vi "UHR-Fleezers Control (host) - Lorentz v3.vi"() -> ()   [LabVIEW 2014] (continued)
      n899 = xnode "Read/Write Control"("FPGA VI Reference In"=w1386, "error in"=w1384, "Invert GI"=w1380, "Invert GI 2"=w1380, "Invert RI"=w1380, "Invert RI 2"=w1380, "Operating Mode"=w1378, "Operating Mode 2"=w1378, "Red Laser Operating Mode"=w1378, "RI Operating Mode 2"=w1378, "P3"=w1410, "I3"=w1411, "D3"=w1412, "Green FB Setpoint"=w1396, "Green FB On/Off"="Green FB On/Off", "Current Out"=w1393, "Green int current ON count adj"="Green int current ON count adj", "Trap Pos FB Monitor T1 or T2"=w1397, "Trap Pos FB Negate Action"=w1398, "Trap Pos. FB Offset Factor"=w1399, "Trap Pos. FB Mult Factor"=w1400, "Force feedback"=FALSE, "AI1 X Scale"=w1402, "Trap Pos to FIFO"=TRUE, "Trap Pos FB Int Count"=w1404, "TTrig Negate Pos"=w1405, "FB Trig Integrate"="FB Trig Integrate", "Diff FB Measurement?"=w1407, "Negate Diff?"="Negate Diff?", "Trap pos. FB Range"=w1381, "Trap Pos. FB Gains"=w1382, "Red FB Setpoint"=w1416, "RI Current Out"=w1420, "P4"=w1422, "I4"=w1423, "D4"=w1424, "Red FB On/Off"="Red FB On/Off", "Dynamic Force FB (Ronen)"=w1383) -> ("error out"=w1385:errorcluster)  [unwired: 1 out]
      n900 = local write "FPGA error out"(w1385) -> ()
    }
    frame #3 {
      # "Initialize more settings. Should stop using event loops to initialize."
      # "What are these?"
      n901 = local write "Offset (nm)"(0.0 ("Offset (nm)")) -> ()
      n902 = local write "Bead Mean (nm)"(0.0 ("Bead Mean (nm)")) -> ()
      n903 = stacked-sequence {
        frame #0 {
          w1428 = T43."empty" ("mode")
          # "Clear external fluorescence triggering FIFO"
          # "APD loop counts"
          # "Fluorescence loop counts (rates)"
          n904 = local read "APD Integration Time (s)"() -> (w1430:dbl)
          n905 = local read "Interlace ON count"() -> (w1431:u16)
          n906 = call "Smart Buffer (DBL) 1.vi"("mode"=w1428) -> ()  [unwired: 5 in, 6 out]
          n907 = call "Smart Buffer (DBL) 2.vi"("mode"=w1428) -> ()  [unwired: 5 in, 6 out]
          n908 = property on="APD Integration Time (s)" class="DigNum (strict)"("Val(Sgnl)"=w1430) -> ()  [unwired: 2 in, 2 out]
          n909 = property on="Interlace ON count" class="DigNum (strict)"("Val(Sgnl)"=w1431) -> ()  [unwired: 2 in, 2 out]
          "Number of APDs" <- 3.0 ("Number of APDs")
        }
        frame #1 {
          # "Number of APDs affects\nAPD DMA transfer"
          # "General settings for all lasers:"
          # "And includes all laser\nON/OFF settings"
          # "Fluorescent lasers settings:"
          # "Blue laser settings:"
          n910 = local read "Laser interlacing mode"() -> (w1433:enum32{"Laser ON", "Laser OFF", "Interlace"})
          n911 = local read "Invert laser interlacing"() -> (w1432:bool)
          n912 = local read "Blue FB On/Off"() -> (w1434:bool)
          n913 = property on="Blue FB On/Off" class="Bool (strict)"("Val(Sgnl)"=w1434) -> ()  [unwired: 2 in, 2 out]
          n914 = property on="Invert laser interlacing" class="Bool (strict)"("Val(Sgnl)"=w1432) -> ()  [unwired: 2 in, 2 out]
          n915 = property on="Laser interlacing mode" class="RadioBtnsControl (strict)"("Val(Sgnl)"=w1433) -> ()  [unwired: 2 in, 2 out]
        }
        frame #2 {
          w1435 = path "C:/Home/Bustamante Lab/Comstock-LabView-Link.udl" ("connection information")
          # "Database link changed by Ronen - not clear if it matter for the program."
          # "Initialize the database connection"
          n916 = disable-structure shown="Disabled" {
            disable-tunnel: [w1438 _] -> w1436
            disable-tunnel: w1435 -> [w1437 _]
            frame Disabled {
              n917 = call-poly <vilib>:"DB Tools Open Connection.vi"("connection information"=w1437) -> ("connection reference"=w1438:T25)  [unwired: 7 in, 1 out]
            }
            frame Enabled {
            }
          }
          "connection reference" <- w1436
          n918 = local write "connection reference"(w1436) -> ()
          n919 = local write "Database link"(w1435) -> ()
        }
        frame #3 {
          # "Load active calibration to fpga"
          n920 = local read "Base N trap periods"() -> (w1440:u32)
          n921 = local read "T1 Osc Enable"() -> (w1439:bool)
          n922 = property on="T1 Osc Enable" class="Bool (strict)"("Val(Sgnl)"=w1439) -> ()  [unwired: 2 in, 2 out]
          n923 = property on="Base N trap periods" class="DigNum (strict)"("Val(Sgnl)"=w1440) -> ()  [unwired: 2 in, 2 out]
        }
      }
    }
    frame #4 {
      # "Set FIFO size and run FPGA"
      n924 = local read "FPGA error out"() -> (w1442:errorcluster)
      n925 = xnode "Invoke Method"("FPGA VI Reference In"=w1443, "error in"=w1442, "Requested Depth"="Trap AI FIFO Depth") -> ("FPGA VI Reference Out"=w1447:T36, "error out"=w1448:errorcluster)  [unwired: 1 out]
      n926 = xnode "Invoke Method"("FPGA VI Reference In"=w1447, "error in"=w1448, "Requested Depth"="Trap Position FIFO Depth") -> ("FPGA VI Reference Out"=w1445:T36, "error out"=w1444:errorcluster)  [unwired: 1 out]
      n927 = xnode "Invoke Method"("FPGA VI Reference In"=w1445, "error in"=w1444) -> ("error out"=w1441:errorcluster)  [unwired: 1 in, 1 out]
      n928 = local write "FPGA error out"(w1441) -> ()
    }
    frame #5 {
      # "Adjust FPGA timing loop phases"
      n929 = flat-sequence "Initial FPGA Loop Relative Phase Adjustment" {
        tunnel: "Initial Phase Adjustment (AI1)" -> [w1482]
        tunnel: "Initial Phase Adjustment (GI)" -> [w1481]
        tunnel: "Initial Phase Adj. (MCL)" -> [w1480]
        tunnel: [w1483] -> w1467
        tunnel: [w1479] -> w1466
        tunnel: "Initial Phase Adjustment (APD Acq)" -> [w1478]
        tunnel: "Initial Phase Adjustment (APD 1 Gate)" -> [w1477]
        tunnel: "Initial Phase Adjustment (Green FB)" -> [w1476]
        tunnel: "Initial Phase Adjustment (GI) 2" -> [w1475]
        tunnel: "Initial Phase Adjustment (APD 2 Gate)" -> [w1474]
        tunnel: "Initial Phase Adjustment (RI)" -> [w1473]
        tunnel: "Initial Phase Adjustment (BI DO)" -> [w1472]
        tunnel: "Initial Phase Adjustment (BI AO)" -> [w1471]
        tunnel: "Initial Phase Adjustment (APD 3 Gate)" -> [w1470]
        tunnel: w1452 -> [w1469]
        tunnel: w1467 -> [w1485]
        tunnel: [w1486] -> w1465
        tunnel: w1466 -> [w1486]
        tunnel: [w1485] -> w1464
        tunnel: w1465 -> [w1490]
        tunnel: w1464 -> [w1489]
        tunnel: [w1487] -> w1451
        frame #0 {
          n930 = local read "FPGA error out"() -> (w1468:errorcluster)
          n931 = xnode "Read/Write Control"("FPGA VI Reference In"=w1469, "error in"=w1468, "Phase count adjustment"=w1482, "Phase count adjustment (GI)"=w1481, "Phase count adjustment (MCL)"=w1480, "Phase Count Adjustment (APD Acq)"=w1478, "Phase count adjustment (APD 1 Gate)"=w1477, "Phase count adjustment (APD 2 Gate)"=w1474, "Phase count adjustment (Green FB)"=w1476, "Phase count adjustment (GI) 2"=w1475, "Phase count adjustment (RI)"=w1473, "Phase count adjustment (BI AO)"=w1471, "Phase count adjustment (BI D)"=w1472, "Phase count adjustment (APD 3 Gate)"=w1470) -> ("FPGA VI Reference Out"=w1479:T36, "error out"=w1483:errorcluster)
        }
        frame #1 {
          n932 = Wait (ms)(milliseconds to wait=u32 100) -> ()  [unwired: 1 out]
        }
        frame #2 {
          w1488 = TRUE
          n933 = xnode "Read/Write Control"("FPGA VI Reference In"=w1490, "error in"=w1489, "+ phase"=w1488, "+ phase (GI)"=w1488, "+ phase (MCL)"=w1488, "+ phase (APD Acq)"=w1488, "+ phase (APD 1 Gate)"=w1488, "+ phase (APD 2 Gate)"=w1488, "+ phase (Green FB)"=w1488, "+ phase (GI) 2"=w1488, "+ phase (RI)"=w1488, "+ phase (BI AO)"=w1488, "+ phase (BI D)"=w1488, "+ phase (APD 3 Gate)"=w1488) -> ("error out"=w1487:errorcluster)  [unwired: 1 out]
        }
      }
      n934 = local write "FPGA error out"(w1451) -> ()
    }
    frame #6 {
      w1504 = 6.0  # clock mult.
      w1503 = 49152000.0  # TCXO frequ.
      w1508 = 6.0  # clock mult.
      w1509 = 49152000.0  # TCXO frequ.
      # "Added by ronen - definition of \nlimit frequencies when using dynamic feedback"
      # "Initialize trap RF synth board and set initial frequencies and amplitudes"
      n935 = local read "FPGA error out"() -> (w1518:errorcluster)
      n936 = call "Initialize RF boards - interlace 3.vi"("error in"=w1518, "FPGA VI Reference In"=w1519) -> ("error out"=w1520:errorcluster, "FPGA VI Reference Out"=w1540:T36)
      n937 = call "set RF board frequency - interlace.vi"("Board 2 Frequency Limits"=w1515, "Board 1 Frequency Limits"=w1496, "error in"=w1520, "FPGA VI Reference In"=w1540, "Board 2 Frequency 3 (MHz)"="BD 2 Frequency 3 (MHz)", "Board 1 Frequency 3 (MHz)"="BD 1 Frequency 3 (MHz)", "Board 2 Frequency 2 (MHz)"="BD 2 Frequency 2 (MHz)", "Board 2 Frequency 1 (MHz)"="BD 2 Frequency 1 (MHz)", "Board 1 Frequency 2 (MHz)"="BD 1 Frequency 2 (MHz)", "Board 1 Frequency 1  (MHz)"="BD 1 Frequency 1 (MHz)") -> ("error out"=w1523:errorcluster, "FPGA VI Reference Out"=w1495:T36)
      n938 = Unbundle By Name(w1496) -> ("Maximum"=w1506:dbl, "Minimum"=w1497:dbl)
      n939 = call "set RF board amplitude - interlace.vi"("Board 2 Amplitude Limits"=w1517, "Board 1 Amplitude Limits"=w1516, "error in"=w1523, "FPGA VI Reference In"=w1495, "Board 2 Amplitude 3 (%)"="BD 2 Amplitude 3 (%)", "Board 1 Amplitude 3 (%)"="BD 1 Amplitude 3 (%)", "Board 2 Amplitude 2 (%)"="BD 2 Amplitude 2 (%)", "Board 2 Amplitude 1 (%)"="BD 2 Amplitude 1 (%)", "Board 1 Amplitude 2 (%)"="BD 1 Amplitude 2 (%)", "Board 1 Amplitude 1 (%)"="BD 1 Amplitude 1 (%)") -> ("error out"=w1492:errorcluster)  [unwired: 1 out]
      n940 = Multiply(x=w1497, y=1000000.0) -> (x*y=w1501:dbl)
      n941 = Multiply(x=w1506, y=1000000.0) -> (x*y=w1511:dbl)
      n942 = Scale By Power Of 2(n=48, x=w1501) -> (x*2^n=w1499:dbl)
      n943 = Subtract(x="BD 1 Frequency 1 (MHz)", y="BD 1 Frequency 2 (MHz)") -> (x-y=w1530:dbl)
      n944 = Subtract(x="BD 2 Frequency 1 (MHz)", y="BD 2 Frequency 2 (MHz)") -> (x-y=w1531:dbl)
      n945 = Scale By Power Of 2(n=48, x=w1511) -> (x*2^n=w1513:dbl)
      n946 = Multiply(x=w1503, y=w1504) -> (x*y=w1505:dbl)
      n947 = Multiply(x=w1509, y=w1508) -> (x*y=w1507:dbl)
      n948 = Square(x=w1531) -> (x^2=w1533:dbl)
      n949 = Square(x=w1530) -> (x^2=w1532:dbl)
      n950 = Divide(x=w1499, y=w1505) -> (x/y=w1500:dbl)
      n951 = Divide(x=w1513, y=w1507) -> (x/y=w1512:dbl)
      n952 = Add(x=w1532, y=w1533) -> (x+y=w1534:dbl)
      n953 = To Unsigned Quad Integer(1:w1500) -> (0:w1493:u64)
      n954 = To Unsigned Quad Integer(1:w1512) -> (0:w1494:u64)
      n955 = Square Root(x=w1534) -> (sqrt(x)=w1535:dbl)
      n956 = local write "Trap Delta (MHz)"(w1535) -> ()
      n957 = xnode "Read/Write Control"("FPGA VI Reference In"=w1495, "error in"=w1492, "FB Max Frequency"=w1494, "FB Min frequency"=w1493) -> ("error out"=w1491:errorcluster)  [unwired: 1 out]
      n958 = local write "FPGA error out"(w1491) -> ()
    }
    frame #7 {
      n959 = local read "FPGA error out"() -> (w1542:errorcluster)
      n960 = flat-sequence {
        tunnel: [w1556] -> w1547
        tunnel: [w1555] -> w1546
        tunnel: w1543 -> [w1549]
        tunnel: w1542 -> [w1548]
        tunnel: [w1560] -> w1545
        tunnel: w1547 -> [w1560]
        tunnel: [w1559] -> w1544
        tunnel: w1546 -> [w1559]
        tunnel: w1545 -> [w1568]
        tunnel: w1544 -> [w1567]
        tunnel: [w1562] -> w1541
        frame #0 {
          n961 = xnode "Read/Write Control"("FPGA VI Reference In"=w1549, "error in"=w1548, "Direct RF Box  Communication"=FALSE) -> ("FPGA VI Reference Out"=w1556:T36, "error out"=w1555:errorcluster)
          n962 = local read "Trap 1 (ON/OFF)"() -> (w1550:bool)
          n963 = local write "Saving..."(FALSE ("Saving Data")) -> ()
          n964 = local write "Stop All"(FALSE ("Stop All")) -> ()
          n965 = local write "Index"(1.0 ("Index")) -> ()
          n966 = property on="Trap 1 ON" class="Bool (strict)"("Value"=w1550) -> ()  [unwired: 2 in, 2 out]
          "Manipulating Trap" <- FALSE ("Manipulating Trap")
        }
        frame #1 {
          n967 = local read "Trap 2 (ON/OFF)"() -> (w1558:bool)
          n968 = Wait (ms)(milliseconds to wait=u32 10) -> ()  [unwired: 1 out]
          n969 = property on="Trap 2 ON" class="Bool (strict)"("Val(Sgnl)"=w1558) -> ()  [unwired: 2 in, 2 out]
        }
        frame #2 {
          n970 = local read "Scan Range (nm)"() -> (w1563:dbl)
          n971 = xnode "Read/Write Control"("FPGA VI Reference In"=w1568, "error in"=w1567, "FPGA Controls  RF Box"=TRUE ("Direct RF Box  Communication")) -> ("error out"=w1562:errorcluster)  [unwired: 1 out]
          n972 = call "Update messages.vi"("Message to add"="UHR-Fleezers ready.", "Old message string"="") -> ("New message string"=w1566:string)
          n973 = local write "Messages"(w1566) -> ()
          n974 = property on="Scan Range (nm)" class="DigNum (strict)"("Val(Sgnl)"=w1563) -> ()  [unwired: 2 in, 2 out]
        }
      }
      n975 = local write "FPGA error out"(w1541) -> ()
    }
    frame #8 {
      w1570 = u32 0
      w1576 = cluster{u32, u32} {16777238, 16777238}
      w1571 = 0.0
      n976 = control-ref of="Piezo trap cursor control"() -> (w1572:refnum<vi>)
      n977 = disable-structure shown="Disabled" {
        disable-tunnel: [w1579 _] -> w1578
        frame Disabled {
          n978 = call "hamilton_controller.vi"("action"=T42."CONNECT") -> ("error out"=w1582:errorcluster)  [unwired: 9 in, 1 out]
          n979 = call "hamilton_controller.vi"("error in"=w1582, "action"=T42."INITIALIZE VALVES") -> ("error out"=w1579:errorcluster)  [unwired: 8 in, 1 out]
        }
        frame Enabled {
        }
      }
      n980 = property class="XYGraph (strict)"(reference=w1572, "XScale.Maximum"=10.0, "XScale.Minimum"=w1571, "YScale.Maximum"=w1571, "YScale.Minimum"=-10.0, "Plot Area Colors"=w1576, "Frame Color"=u32 9868950, "XScale.GridColors"=w1576, "YScale.GridColors"=w1576, "Cursor.Cursor Color"=u32 16711680, "Active Cursor"=w1570, "Cursor.CursorMode"=w1570) -> ()  [unwired: 1 in, 2 out]
    }
    frame #9 {
      # "Wait 5 s for all the event loops still being executed to finish."
      n981 = Wait (ms)(milliseconds to wait=u32 5000) -> ()  [unwired: 1 out]
      n982 = local read "FPGA error out"() -> (w1584:errorcluster)
    }
    frame #10 {
      # "Initialize Serial communication with Arduino, and clear the buffer first"
      n983 = Unbundle By Name("Serial Settings for arduino") -> ("baud rate"=w1599:u32, "data bits"=w1598:u16, "parity"=w1597:enum16{"None", "Odd", "Even", "Mark", "Space"}, "stop bits"=w1596:u16, "flow control"=w1595:u16, "Time out (ms)"=w1593:u32)
      n984 = call-poly "VISA Configure Serial Port"("VISA resource name"="VISA resource name", "timeout (10sec)"=w1593, "Enable Termination\nChar (T)"=FALSE, "baud rate (9600)"=w1599, "data bits (8)"=w1598, "parity (0:none)"=w1597, "error in (no error)"="Serial Error in", "stop bits (10: 1 bit)"=w1596, "flow control (0:none)"=w1595) -> ("VISA resource name out"=w1589:refnum<visa-resource-name>, "error out"=w1588:errorcluster)  [unwired: 5 in]
      n985 = VISA Clear(VISA resource name=w1589, error in (no error)=w1588) -> (VISA resource name out=w1586:refnum<visa-resource-name>, error out=w1587:errorcluster)
    }
  }
  n986 = node-c288() -> (w33:T37)  [unwired: 4 out]
  n987 = disable-structure shown="Disabled" {
    frame Disabled {
      n988 = while "Duncan's play event loop" {
        stop <- w1602 stop-if-true
        n989 = Create User Event(user event datatype=TRUE ("Boolean")) -> (user event=w1603:refnum<user-event>)  [unwired: 1 in, 1 out]
        n990 = Create User Event(user event datatype=TRUE ("Boolean")) -> (user event=w1609:refnum<user-event>)  [unwired: 1 in, 1 out]
        n991 = global write "Global for fluorescence simulation mean (30 samples), (power series).vi" "Red Signal"(w1603) -> ()
        n992 = global write "Global for fluorescence simulation mean (30 samples), (power series).vi" "Green Signal"(w1609) -> ()
        n993 = register-events(w1609, w1603) -> (reference out=w1608:refnum<event-registration>)  [unwired: 2 in, 1 out]
        n994 = event shown="[1] \"Start assembly line\": Value Change" {
          selector: w1608 -> [_ _ _ _]
          dyn-events: _ -> [_ _ _ _]
          timeout: 100 -> [_ _ _ _]
          event Timeout {
            n995 = event-data() -> ()  [unwired: 1 in, 2 out]
          }
          event "Start assembly line": Value Change {
            n996 = event-data() -> ("OldVal"=w1611:bool)  [unwired: 1 in, 4 out]
            n997 = case shown="True" w1611 {
              selector: w1611 -> [_ w1612]
              frame False {
              }
              frame True {
                n998 = property on="Move to Position 3" class="Bool"("Val(Sgnl)"=w1612) -> ()  [unwired: 2 in, 2 out]
                n999 = case shown="1" "Numeric" {
                  frame 0, Default {
                  }
                  frame 1 {
                    n1000 = property on="Green Laser ON" class="Bool (strict)"("Val(Sgnl)"=TRUE ("Value (Signaling)")) -> ()  [unwired: 2 in, 2 out]
                  }
                  frame 2 {
                    n1001 = property on="Red Laser ON" class="Bool (strict)"("Val(Sgnl)"=TRUE) -> ()  [unwired: 2 in, 2 out]
                  }
                }
              }
            }
          }
          event User Event {
            n1002 = event-data() -> ("Boolean"=w1616:bool)  [unwired: 1 in, 3 out]
            "Green Fluorophore" <- w1616
            n1003 = property on="Start assembly line" class="Bool"("Val(Sgnl)"=w1616) -> ()  [unwired: 2 in, 2 out]
          }
          event User Event {
            n1004 = event-data() -> ("Boolean"=w1617:bool)  [unwired: 1 in, 3 out]
            "Red Fluorophore" <- w1617
            n1005 = property on="Start assembly line" class="Bool"("Val(Sgnl)"=w1617) -> ()  [unwired: 2 in, 2 out]
          }
        }
        n1006 = property on="Get Fluorophore" class="Bool (strict)"("Val(Sgnl)"="Get Fluorophore") -> ()  [unwired: 2 in, 2 out]
        n1007 = Wait (ms)(milliseconds to wait=u32 100) -> ()  [unwired: 1 out]
        n1008 = local read "Stop All"() -> (w1601:bool)
        n1009 = Or(x=w1601, y="stop") -> (x .or. y?=w1602:bool)
      }
    }
    frame Enabled {
    }
  }
  n1010 = timed-loop "Rough control of MCL mirror stage (debugging)" {
    tunnel: [w1620] -> w74
    timing: w33 -> [_]
    timing-out: [_] -> w32
    tunnel: w24 -> [w1618]
    stop <- w1620 stop-if-true
    n1011 = node-c288() -> ()  [unwired: 2 out]
    n1012 = case shown="1" "MCL Mode" {
      tunnel: w1618 -> [_ w1623 w1670]
      frame 0, Default {
      }
      frame 1 {
        n1013 = node-c288() -> (w1625:T37)  [unwired: 4 out]
        n1014 = timed-loop "Oscillate MCL mirror" {
          timing: w1625 -> [_]
          timing-out: [_] -> w1624
          tunnel: w1623 -> [w1626]
          i -> [w1664]
          stop <- w1627 stop-if-true
          n1015 = node-c288() -> (w1663:i64)  [unwired: 1 out]
          n1016 = Multiply(x="AO1", y=32767.0) -> (x*y=w1659:dbl)
          n1017 = Multiply(x="AO2", y=32767.0) -> (x*y=w1654:dbl)
          n1018 = Divide(x=w1659, y=10.0) -> (x/y=w1660:dbl)
          n1019 = Divide(x=w1654, y=10.0) -> (x/y=w1655:dbl)
          n1020 = To Word Integer(number=w1660) -> (16bit integer=w1652:i16)
          n1021 = To Word Integer(number=w1655) -> (16bit integer=w1651:i16)
          n1022 = Divide(x=w1663, y=i64 1000) -> (x/y=w1634:dbl)
          n1023 = Multiply(x=w1634, y=w1664) -> (x*y=w1645:dbl)
          n1024 = Multiply(x="Osc. freq. (Hz) 2", y=6.283185307179586) -> (x*y=w1646:dbl)
          n1025 = Multiply(x=w1646, y=w1645) -> (x*y=w1644:dbl)
          n1026 = Sine(x=w1644) -> (sin(x)=w1643:dbl)
          n1027 = Multiply(x=w1643, y="Osc. amp. (V)") -> (x*y=w1641:dbl)
          n1028 = Add(x=w1641, y="Osc. center (V)") -> (x+y=w1639:dbl)
          n1029 = Divide(x=w1639, y=10.0) -> (x/y=w1637:dbl)
          n1030 = Multiply(x=w1637, y=32767.0) -> (x*y=w1632:dbl)
          n1031 = Select(t=w1632, s="Scan axis", f=w1652) -> (s? t:f=w1650:dbl)
          n1032 = Select(t=w1651, s="Scan axis", f=w1632) -> (s? t:f=w1649:dbl)
          n1033 = local read "MCL Mode"() -> (w1631:u16)
          n1034 = Not Equal?(x=w1631, y=u16 1) -> (x != y?=w1628:bool)
          n1035 = local read "Stop All"() -> (w1629:bool)
          n1036 = xnode "Read/Write Control"("FPGA VI Reference In"=w1626, "AO1"=w1650, "AO2"=w1649) -> ()  [unwired: 1 in, 2 out]
          n1037 = Compound Arithmetic op=OR(w1629, w1628) -> (w1627:bool)
          n1038 = node-c288() -> ()  [unwired: 2 out]
        }
        n1039 = node-c288(w1624) -> ()  [unwired: 1 out]
      }
      frame 2 {
        n1040 = case shown="True" "Start Scan" {
          tunnel: w1670 -> [_ w1672]
          frame False {
          }
          frame True {
            n1041 = Subtract(x="End (V)", y="Begin (V)") -> (x-y=w1679:dbl)
            n1042 = Decrement(x="N Points") -> (x-1=w1678:dbl)
            n1043 = Divide(x=w1679, y=w1678) -> (x/y=w1676:dbl)
            n1044 = for {
              N: "N Points" -> [_]
              tunnel: "Begin (V)" -> [w1695]
              tunnel: [w1687] -> w1682 mode=indexing
              tunnel: w1676 -> [w1686]
              tunnel: [w1684] -> w1675 mode=indexing
              tunnel: w1672 -> [w1683]
              i -> [w1694]
              n1045 = Multiply(x=w1686, y=w1694) -> (x*y=w1693:dbl)
              n1046 = Add(x=w1695, y=w1693) -> (x+y=w1690:dbl)
              n1047 = local read "Scan axis"() -> (w1685:bool)
              n1048 = local read "AO1"() -> (w1692:dbl)
              n1049 = local read "AO2"() -> (w1691:dbl)
              n1050 = Select(t=w1690, s=w1685, f=w1692) -> (s? t:f=w1689:dbl)
              n1051 = Select(t=w1691, s=w1685, f=w1690) -> (s? t:f=w1688:dbl)
              n1052 = flat-sequence {
                tunnel: w1689 -> [w1699]
                tunnel: w1688 -> [w1698]
                tunnel: w1683 -> [w1696]
                tunnel: [w1709] -> w1687
                tunnel: [w1708] -> w1684
                frame #0 {
                  w1702 = 10.0 ("y")
                  w1697 = 32767.0 ("y")
                  n1053 = Multiply(x=w1699, y=w1697) -> (x*y=w1705:dbl)
                  n1054 = Multiply(x=w1698, y=w1697) -> (x*y=w1703:dbl)
                  n1055 = Divide(x=w1705, y=w1702) -> (x/y=w1706:dbl)
                  n1056 = Divide(x=w1703, y=w1702) -> (x/y=w1704:dbl)
                  n1057 = To Word Integer(number=w1706) -> (16bit integer=w1700:i16)
                  n1058 = To Word Integer(number=w1704) -> (16bit integer=w1701:i16)
                  n1059 = xnode "Read/Write Control"("FPGA VI Reference In"=w1696, "AO1"=w1700, "AO2"=w1701) -> ()  [unwired: 1 in, 2 out]
                }
                frame #1 {
                  n1060 = Wait (ms)(milliseconds to wait="DAQ Delay (ms)") -> ()  [unwired: 1 out]
                }
                frame #2 {
                  n1061 = local read "Slow mean"() -> (w1709:dbl)
                  n1062 = local read "Sigma"() -> (w1708:dbl)
                }
              }
            }
            n1063 = Bundle("Begin (V)"="Begin (V)", w1676, w1682) -> (→"MCL Scan":cluster{"Begin (V)":dbl, dbl, dbl[]})  [unwired: 1 out]
            n1064 = Bundle("Begin (V)"="Begin (V)", w1676, w1675) -> (→"MCL Scan 2":cluster{"Begin (V)":dbl, dbl, dbl[]})  [unwired: 1 out]
          }
        }
      }
    }
    n1065 = local read "Stop All"() -> (w1620:bool)
    n1066 = node-c288() -> ()  [unwired: 2 out]
  }
  n1067 = node-c288(2 ("Processor")) -> (w65:T37)  [unwired: 3 out]
  n1068 = timed-loop "Basic control parameters (all FPGA settings, other basic controls)" {
    shift-right: [w1717] -> _
    shift-left: errorcluster {"status"=FALSE, "code"=0, "source"=""} ("error out") -> [_]
    tunnel: [w1716] -> _
    timing: w65 -> [_]
    timing-out: [_] -> w64
    tunnel: w46 -> [w1715]
    tunnel: w42 -> [w1714]
    tunnel: w41 -> [w1713]
    tunnel: w40 -> [w1712]
    tunnel: w39 -> [w1711]
    tunnel: w24 -> [w1710]
    stop <- w1716 stop-if-true
    n1069 = node-c288() -> ()  [unwired: 2 out]
    n1070 = event shown="[87] \"Cursor control.X\", \"Cursor control.Y\": Value Change" {
      selector: _ -> [_ _ _ _ _ _ _ _ _ _ _ _ _ _ _ _ _ _ _ _ _ _ _ _ _ _ _ _ _ _ _ _ _ _ _ _ _ _ _ _ _ _ _ _ _ _ _ _ _ _ _ _ _ _ _ _ _ _ _ _ _ _ _ _ _ _ _ _ _ _ _ _ _ _ _ _ _ _ _ _ _ _ _ _ _ _ _ _]
      dyn-events: _ -> [_ _ _ _ _ _ _ _ _ _ _ _ _ _ _ _ _ _ _ _ _ _ _ _ _ _ _ _ _ _ _ _ _ _ _ _ _ _ _ _ _ _ _ _ _ _ _ _ _ _ _ _ _ _ _ _ _ _ _ _ _ _ _ _ _ _ _ _ _ _ _ _ _ _ _ _ _ _ _ _ _ _ _ _ _ _ _ _]
      timeout: _ -> [_ _ _ _ _ _ _ _ _ _ _ _ _ _ _ _ _ _ _ _ _ _ _ _ _ _ _ _ _ _ _ _ _ _ _ _ _ _ _ _ _ _ _ _ _ _ _ _ _ _ _ _ _ _ _ _ _ _ _ _ _ _ _ _ _ _ _ _ _ _ _ _ _ _ _ _ _ _ _ _ _ _ _ _ _ _ _ _]
      tunnel: [w1757 _ _ _ w1784 _ _ _ _ _ _ _ w1890 _ _ w1977 w1979 w1986 w1988 w2058 _ w2100 w2126 w2154 w2179 w2206 w2232 w2261 _ w2266 w2360 w2364 w2401 _ w2464 w2467 w2470 w2480 w2483 _ w2490 _ _ _ _ _ _ _ _ _ _ _ _ _ _ _ _ _ _ _ _ w2987 _ _ _ _ w3024 _ _ _ _ _ _ _ _ _ _ _ _ _ _ _ _ _ _ w3305 _ _] -> w1717
      tunnel: [_ _ _ _ _ _ _ _ _ _ w1869 _ _ _ _ _ _ _ _ _ _ _ _ _ _ _ _ _ _ _ _ _ _ _ _ _ _ _ _ _ _ _ _ _ _ _ _ _ _ _ _ _ _ _ _ _ _ _ _ _ _ _ _ _ _ _ _ _ _ _ _ _ _ _ _ _ _ _ _ _ _ _ _ _ _ _ _ _] -> w1716
      tunnel: [_ _ _ _ _ _ _ _ "Round T1 X" _ _ _ _ _ _ _ _ _ _ _ _ _ _ _ _ _ _ _ _ _ _ _ _ _ _ _ _ _ _ _ _ _ _ _ _ _ _ _ _ _ _ _ _ _ _ _ _ _ _ _ _ _ _ _ _ _ _ _ _ _ _ _ _ _ _ _ _ _ _ _ _ _ _ _ _ _ _ _] -> _
      tunnel: [_ _ _ "Adjust Scale\nto Mean" _ _ _ _ _ _ _ _ _ _ _ _ _ _ _ _ _ _ _ _ _ _ _ _ _ "Test ttrig" _ _ _ _ _ _ _ _ _ _ _ _ _ _ _ _ _ _ _ _ _ w2734 w2798 w2845 w2894 _ _ _ _ _ _ _ _ _ _ _ _ _ _ _ _ _ _ _ _ _ _ _ _ _ _ _ _ _ _ _ _ _] -> _
      tunnel: [_ _ _ _ _ _ _ _ _ "Round T2 X" _ "Delayed Interlace Start" _ _ _ _ _ _ _ _ _ _ _ _ _ _ _ _ _ _ _ _ _ _ _ _ _ _ _ _ _ _ _ _ _ _ _ _ _ _ _ _ _ _ _ _ _ _ _ _ _ _ _ _ _ _ _ _ _ _ _ _ _ _ _ _ _ _ _ _ _ _ _ _ _ _ _ _] -> _
      tunnel: w1715 -> [_ _ _ _ _ _ _ _ _ _ _ _ _ _ _ _ _ _ _ _ _ _ _ _ _ _ _ _ _ _ _ _ _ _ _ _ _ _ _ _ _ _ _ _ _ _ _ w2704 w2712 w2719 w2725 w2733 _ _ w2893 _ _ _ _ _ _ _ _ _ _ _ _ _ _ _ _ _ _ _ _ _ _ _ _ _ _ _ _ _ _ _ _ _]
      tunnel: w1714 -> [_ _ _ _ _ _ _ _ _ _ _ _ _ _ _ _ _ _ _ _ _ _ _ _ _ _ _ _ _ _ _ _ _ _ _ _ _ _ _ _ _ _ _ _ _ w2591 _ _ _ _ _ _ w2797 _ _ w2900 _ w2912 _ w2928 _ _ _ _ _ _ _ _ _ _ _ _ _ _ _ _ _ _ _ _ _ _ _ _ _ _ _ _]
      tunnel: w1713 -> [_ _ _ _ _ _ _ _ _ _ _ _ _ _ _ _ _ _ _ _ _ _ _ _ _ _ _ _ _ _ _ _ _ _ _ _ _ _ _ _ _ _ _ _ _ _ _ _ _ _ _ _ _ _ _ _ _ _ _ _ _ _ _ _ _ _ _ _ _ _ _ _ _ _ _ _ _ _ _ _ _ _ _ _ _ _ _ _]
      tunnel: w1712 -> [_ _ _ _ _ _ _ _ _ _ _ _ _ _ _ _ _ _ _ _ _ _ _ _ _ _ _ _ _ _ _ _ _ _ _ _ _ _ _ _ _ w2501 _ _ _ _ _ _ _ _ _ _ _ w2844 _ _ w2906 _ w2920 _ w2954 _ _ _ _ _ _ _ _ _ _ _ _ _ _ _ _ _ _ _ _ _ _ _ _ _ _ _]
      tunnel: w1711 -> [_ _ _ _ _ _ _ _ _ _ _ _ _ _ _ _ _ _ _ _ _ _ _ _ _ _ _ _ _ _ _ _ _ _ _ _ _ _ _ _ _ _ _ _ _ _ _ _ _ _ _ _ _ _ _ _ _ _ _ _ _ _ _ _ _ _ _ _ _ _ _ _ _ _ _ _ _ _ _ _ _ _ _ _ _ _ _ _]
      tunnel: w1710 -> [w1720 _ _ _ w1783 _ w1809 _ _ _ _ _ w1881 _ _ w1961 w1978 w1985 w1987 w2023 _ w2089 w2124 w2136 w2161 w2189 w2209 w2237 w2262 w2264 w2268 w2361 w2365 _ w2461 w2465 w2468 w2478 w2481 _ w2489 _ _ _ _ _ _ _ _ _ _ _ _ _ _ _ _ _ _ _ _ w2980 _ w3001 _ w3008 w3023 _ w3030 w3057 w3064 w3080 w3088 _ w3099 _ w3143 _ _ w3197 w3228 w3232 w3240 _ w3304 _ w3318 w3337]
      tunnel: [_ _ _ _ _ _ _ _ _ _ w1868 _ _ _ _ _ _ _ _ _ _ _ _ _ _ _ _ _ _ _ _ _ _ _ _ _ _ _ _ _ _ _ w2579 w2583 w2587 _ _ _ _ _ _ _ _ _ _ _ _ _ _ _ _ _ _ _ _ _ _ _ _ _ _ _ _ _ _ _ _ _ _ _ _ _ _ _ _ _ _ _] -> _
      event "AI Count (ticks)", "Sets to FIFO (Traps)", "Save ave N", "FPGA Ave.", "# Samples/channel", "N sets to save": Value Change {
        # "RG 18-01-16 Increased amount of elements to read for trap position, to add x and y for piezo trap"
        # "So that if 'Save ave N' is updated, the AOD scanning code updates too."
        n1071 = event-data() -> ()  [unwired: 6 out]
        n1072 = local read "AI Count (ticks)"() -> (w1741:u16)
        n1073 = Divide(x=40000000.0, y=w1741) -> (x/y=w1733:dbl)
        "AI rate (Hz)" <- w1733
        "Ave. Rate (Hz)" <- w1733
        n1074 = Reciprocal(x=w1733) -> (1/x=→"Ave. Period (s)":dbl)
        n1075 = Unbundle By Name("Sets to FIFO (Traps)") -> ("Set 1"=w1724:bool, "Set 2"=w1723:bool, "Set 3"=w1722:bool)
        n1076 = Divide(x=w1733, y="N Acq Sets (Traps + Fl.)") -> (x/y=w1754:dbl)
        "Data Rate (Hz)" <- w1754
        n1077 = Reciprocal(x=w1754) -> (1/x=→"Data Period (s)":dbl)
        n1078 = Boolean To (0,1)(Boolean="Sets to FIFO (Traps)") -> (0, 1=w1749:cluster{"Set 1":i16, "Set 2":i16, "Set 3":i16})
        n1079 = xnode "Read/Write Control"("FPGA VI Reference In"=w1720, "ai count"=w1741, "Set 1"=w1724, "Set 2"=w1723, "Set 3"=w1722, "N of AI1 Int Acq Sets"="N Acq Sets (Traps + Fl.)") -> ("error out"=w1757:errorcluster)  [unwired: 1 in, 1 out]
        n1080 = Cluster To Array(cluster=w1749) -> (array=w1748:i16[])
        n1081 = local read "Save ave N"() -> (w1753:dbl)
        n1082 = To Unsigned Long Integer(number=w1748) -> (unsigned 32bit integer=w1730:u32[])
        n1083 = local read "Scan steps (AOD)"() -> (w1750:u64)
        n1084 = Multiply(x=w1741, y="N Acq Sets (Traps + Fl.)") -> (x*y=w1739:u16)
        n1085 = Add Array Elements(numeric array=w1730) -> (sum=w1742:u32)
        "Trap Sets" <- w1742
        n1086 = Divide(x=w1754, y=w1753) -> (x/y=w1752:dbl)
        "Save Data Rate (Hz)" <- w1752
        n1087 = Reciprocal(x=w1752) -> (1/x=→"Save Data Period (s)":dbl)
        n1088 = property on="Scan steps (AOD)" class="DigNum (strict)"("Val(Sgnl)"=w1750) -> ()  [unwired: 2 in, 2 out]
        n1089 = Multiply(x=w1739, y="# Samples/trap") -> (x*y=w1737:u32)
        "Counts/DMA" <- w1737
        n1090 = property on="Trap Disp. Downsample" class="DigNum (strict)"("Maximum"="# Samples/trap") -> ()  [unwired: 2 in, 2 out]
        n1091 = Multiply(x=w1742, y="# Samples/trap") -> (x*y=w1731:u32)
        "# Samples/channel" <- w1731
        n1092 = Multiply(x=w1731, y=u32 8) -> (x*y=→"Trap AI Elements/DMA read":u32)
        n1093 = local read "APD Int. Count"() -> (w1738:u32)
        n1094 = Multiply(x=w1731, y=u32 5) -> (x*y=→"Trap Pos Elements/DMA read":u32)
        n1095 = Divide(x=w1737, y=w1738) -> (x/y=w1728:dbl)
        "APD Samples/FIFO Acq." <- w1728
        n1096 = Divide(x=w1737, y=40000000.0) -> (x/y=w1735:dbl)
        "DMA Update Period (s)" <- w1735
        n1097 = local read "Number of APDs"() -> (w1721:u8)
        n1098 = Multiply(x=w1721, y=w1728) -> (x*y=→"APD Elements/DMA read":dbl)
        n1099 = property on="APD Disp. Downsample" class="DigNum (strict)"("Maximum"=w1728) -> ()  [unwired: 2 in, 2 out]
        n1100 = local read "N sets to save"() -> (w1747:u32)
        n1101 = Multiply(x=w1735, y=w1747) -> (x*y=→"Total Time (s) 2":dbl)
        "FPGA Averaging" <- FALSE ("FPGA Averaging")
      }
      event "Remove Offset": Value Change {
        n1102 = event-data() -> ()  [unwired: 7 out]
        n1103 = local write "Remove Offset"(FALSE ("Remove Offset")) -> ()
        n1104 = local read "Bead Mean (nm)"() -> (w1759:dbl)
        n1105 = local read "Offset (nm)"() -> (w1760:dbl)
        n1106 = Add(x=w1759, y=w1760) -> (x+y=w1758:dbl)
        n1107 = local write "Offset (nm)"(w1758) -> ()
      }
      event "Detector Type": Value Change {
        n1108 = event-data() -> ()  [unwired: 7 out]
        n1109 = local read "AI labels"() -> (w1764:string[])
        n1110 = property on="High Res. Display" class="Ring (strict)"("Strings []"=w1764) -> ()  [unwired: 2 in, 2 out]
        n1111 = Build Array (concatenate)(w1764, "none") -> (w1765:string[])
        n1112 = property on="FFT 1 Choice 1" class="Ring (strict)"("Strings []"=w1765) -> ()  [unwired: 2 in, 2 out]
        n1113 = property on="FFT 1 Choice 2" class="Ring (strict)"("Strings []"=w1765) -> ()  [unwired: 2 in, 2 out]
        n1114 = property on="FFT 2 Choice 1" class="Ring (strict)"("Strings []"=w1765) -> ()  [unwired: 2 in, 2 out]
        n1115 = property on="FFT 2 Choice 2" class="Ring (strict)"("Strings []"=w1765) -> ()  [unwired: 2 in, 2 out]
        n1116 = Bundle("APD 1", "APD 2", "APD 3") -> (w1768:cluster{string, string, string})  [unwired: 1 out]
        n1117 = Cluster To Array(cluster=w1768) -> (array=w1766:string[])
        n1118 = Build Array (concatenate)(w1766, w1765) -> (w1770:string[])
        n1119 = Array Size(array=w1770) -> (size(s)=w1762:i32)
        n1120 = property on="Signals to Plot" class="LstBox (strict)"("Item Names"=w1770) -> ()  [unwired: 2 in, 2 out]
        n1121 = property on="Signals to Plot" class="LstBox (strict)"("Number of Rows"=w1762) -> ()  [unwired: 2 in, 2 out]
        n1122 = property on="All Signals" class="WFChart (strict)"("LegNumRows"=w1762) -> ()  [unwired: 2 in, 2 out]
      }
      event "Adjust Scale\nto Mean": Value Change {
        n1123 = event-data() -> ()  [unwired: 7 out]
        n1124 = local read "APD rates cluster"() -> (w1773:T1)
        n1125 = Unbundle By Name(w1773) -> ("APD 1 Rate (Hz)"=w1772:dbl)
        n1126 = Multiply(x=1000.0, y="Above (kHz)") -> (x*y=w1779:dbl)
        n1127 = Multiply(x=1000.0, y="Below (kHz)") -> (x*y=w1777:dbl)
        n1128 = Add(x=w1779, y=w1772) -> (x+y=w1774:dbl)
        n1129 = Subtract(x=w1772, y=w1777) -> (x-y=w1775:dbl)
        n1130 = property on="APD Chart" class="WFChart (strict)"("YScale.Minimum"=w1775) -> ()  [unwired: 2 in, 2 out]
        n1131 = property on="APD Chart" class="WFChart (strict)"("YScale.Maximum"=w1774) -> ()  [unwired: 2 in, 2 out]
      }
      event "Phase adj. (AI1)", "+ phase (AI1)", "- phase (AI1)": Value Change {
        n1132 = event-data() -> ()  [unwired: 7 out]
        n1133 = Negate(x="Phase adj. (AI1)") -> (-x=w1791:i16)
        n1134 = Select(t=w1791, s="- phase (AI1)", f="Phase adj. (AI1)") -> (s? t:f=w1790:i16)
        n1135 = xnode "Read/Write Control"("FPGA VI Reference In"=w1783, "Phase count adjustment"=w1790) -> ("FPGA VI Reference Out"=w1789:T36, "error out"=w1788:errorcluster)  [unwired: 2 in]
        n1136 = Or(x="- phase (AI1)", y="+ phase (AI1)") -> (x .or. y?=w1785:bool)
        n1137 = xnode "Read/Write Control"("FPGA VI Reference In"=w1789, "error in"=w1788, "+ phase"=w1785) -> ("error out"=w1784:errorcluster)  [unwired: 1 in, 1 out]
      }
      event "Signals to Plot": Double Click {
        w1803 = u32 9868950 ("Color Box")
        n1138 = event-data() -> ("Row"=w1794:i32)  [unwired: 9 out]
        n1139 = property on="All Signals" class="WFChart (strict)"("Active Plot"=w1794) -> (error out=w1793:errorcluster)  [unwired: 2 in, 1 out]
        n1140 = property on="All Signals" class="WFChart (strict)" props=["Plot", "Plot Color", "Plot", "Visible?"](error in=w1793) -> (error out=w1796:errorcluster, "Plot.Visible?"=w1795:bool)  [unwired: 1 in, 2 out]
        n1141 = Select(t=FALSE ("Plot.Visible"), s=w1795, f=TRUE ("Plot.Visible")) -> (s? t:f=w1798:bool)
        n1142 = property on="All Signals" class="WFChart (strict)"(error in=w1796, "Plot.Visible?"=w1798) -> (error out=w1797:errorcluster)  [unwired: 1 in, 1 out]
        n1143 = property on="All Signals" class="WFChart (strict)"(error in=w1797) -> (error out=w1799:errorcluster, "Plot.Plot Color"=w1800:u32)  [unwired: 1 in, 1 out]
        n1144 = property on="Signals to Plot" class="LstBox (strict)"(error in=w1799, "Active Row"=w1794) -> (error out=w1804:errorcluster)  [unwired: 1 in, 1 out]
        n1145 = Select(t=w1800, s=w1798, f=u32 0) -> (s? t:f=w1805:u32)
        n1146 = property on="Signals to Plot" class="LstBox (strict)"(error in=w1804, "CellFontColor"=w1805, "SelColor"=w1803, "CellBG"=w1803, "CellFontSize"=u32 20 ("Active Row:Cell Font:Size"), "CellFontBold"=TRUE ("Active Row:Cell Font:Bold")) -> ()  [unwired: 1 in, 2 out]
      }
      event "BD 1 Frequency 1 (MHz)", "BD 1 Frequency 2 (MHz)", "BD 1 Frequency 3 (MHz)", "BD 2 Frequency 1 (MHz)", "BD 2 Frequency 2 (MHz)", "BD 2 Frequency 3 (MHz)", "Trap Delta (MHz)", "Update all trap values": Value Change {
        # "This is so you can set trap frequencies\nvia local variables and then update\nall at once"
        n1147 = event-data() -> ("CtlRef"=w1813:refnum<vi>)  [unwired: 6 out]
        n1148 = control-ref of="Trap Delta (MHz)"() -> (w1812:refnum<vi>)
        n1149 = Equal?(x=w1812, y=w1813) -> (x = y?=w1811:bool)
        n1150 = local write "Update all trap values"(FALSE ("Update all trap values")) -> ()
        n1151 = case shown="False" "Oscillate Set 1" {
          tunnel: w1811 -> [w1827 _]
          tunnel: w1809 -> [w1825 _]
          frame False {
            n1152 = local read "BD 1 Frequency 2 (MHz)"() -> (w1823:dbl)
            n1153 = case shown="False" "Symmetric?" {
              tunnel: "Trap Delta (MHz)" -> [w1849 w1856]
              tunnel: [w1850 w1854] -> w1815
              tunnel: [w1848 w1851] -> w1817
              tunnel: w1823 -> [w1850 _]
              frame False {
                n1154 = Subtract(x=w1850, y=w1849) -> (x-y=w1848:dbl)
              }
              frame True {
                w1853 = 75
                n1155 = Divide(x=w1856, y=2.0) -> (x/y=w1852:dbl)
                n1156 = Add(x=w1852, y=w1853) -> (x+y=w1854:dbl)
                n1157 = Subtract(x=w1853, y=w1852) -> (x-y=w1851:dbl)
              }
            }
            n1158 = local read "BD 1 Frequency 1 (MHz)"() -> (w1818:dbl)
            n1159 = Not(x="Symmetric?") -> (.not. x?=w1821:bool)
            n1160 = And(x=w1821, y="move Con X?") -> (x .and. y?=w1819:bool)
            n1161 = Subtract(x=w1818, y=w1817) -> (x-y=w1816:dbl)
            n1162 = Select(t=w1817, s=w1827, f=w1818) -> (s? t:f=w1826:dbl)
            n1163 = local read "Y RF Frequency Limits (MHz)"() -> (w1828:T24)
            n1164 = case shown="True" w1819 {
              tunnel: w1816 -> [_ w1847]
              frame False {
              }
              frame True {
                n1165 = property on="AOM X Cal (nm/MHz)" class="DigNum (strict)"() -> ("Value"=w1846:dbl)  [unwired: 2 in, 2 out]
                n1166 = property on="MCL Step Position Ratio" class="DigNum (strict)"() -> ("Value"=w1840:dbl)  [unwired: 2 in, 2 out]
                n1167 = Compound Arithmetic op=MULTIPLY(w1847, w1846, w1840) -> (w1845:dbl)
                n1168 = property on="MCL X Cal (nm/V)" class="DigNum (strict)"() -> ("Value"=w1844:dbl)  [unwired: 2 in, 2 out]
                n1169 = Divide(x=w1845, y=w1844) -> (x/y=w1843:dbl)
                n1170 = property on="AO2" class="Slide (strict)"() -> ("Value"=w1842:dbl)  [unwired: 2 in, 2 out]
                n1171 = Add(x=w1843, y=w1842) -> (x+y=w1841:dbl)
                n1172 = property on="AO2" class="Slide (strict)"("Val(Sgnl)"=w1841) -> ()  [unwired: 2 in, 2 out]
              }
            }
            n1173 = local read "X RF Frequency Limits (MHz)"() -> (w1829:T24)
            n1174 = local write "BD 1 Frequency 1 (MHz)"(w1826) -> ()
            n1175 = local read "BD 1 Frequency 3 (MHz)"() -> (w1838:dbl)
            n1176 = local read "BD 2 Frequency 1 (MHz)"() -> (w1832:dbl)
            n1177 = local read "BD 2 Frequency 2 (MHz)"() -> (w1831:dbl)
            n1178 = local read "BD 2 Frequency 3 (MHz)"() -> (w1839:dbl)
            n1179 = call "set RF board frequency - interlace.vi"("Board 2 Frequency Limits"=w1828, "Board 1 Frequency Limits"=w1829, "FPGA VI Reference In"=w1825, "Board 2 Frequency 3 (MHz)"=w1839, "Board 1 Frequency 3 (MHz)"=w1838, "Board 2 Frequency 2 (MHz)"=w1831, "Board 2 Frequency 1 (MHz)"=w1832, "Board 1 Frequency 2 (MHz)"=w1815, "Board 1 Frequency 1  (MHz)"=w1826) -> ()  [unwired: 1 in, 2 out]
            n1180 = Subtract(x=w1832, y=w1831) -> (x-y=w1836:dbl)
            n1181 = local write "BD 1 Frequency 2 (MHz)"(w1815) -> ()
            n1182 = Subtract(x=w1826, y=w1815) -> (x-y=w1837:dbl)
            n1183 = Square(x=w1836) -> (x^2=w1834:dbl)
            n1184 = Square(x=w1837) -> (x^2=w1835:dbl)
            n1185 = Add(x=w1835, y=w1834) -> (x+y=w1833:dbl)
            n1186 = Square Root(x=w1833) -> (sqrt(x)=w1830:dbl)
            n1187 = property on="Initial delta (MHz)" class="DigNum (strict)"("Val(Sgnl)"=w1830) -> ()  [unwired: 2 in, 2 out]
            n1188 = local write "Trap Delta (MHz)"(w1830) -> ()
          }
          frame True {
          }
        }
      }
      event "manual raster set": Value Change {
        n1189 = event-data() -> ()  [unwired: 7 out]
        n1190 = flat-sequence {
          frame #0 {
            n1191 = Replace Array Subset(array=u32[] [0] ("Index Values"), new element="manual raster set", index=0) -> (w1857:u32[])
            n1192 = property on="Saved AOD Raster Scan Parameter Sets" class="Arr (strict)"("Index Values"=w1857) -> ()  [unwired: 2 in, 2 out]
          }
          frame #1 {
            n1193 = property on="Load parameters" class="Bool (strict)"("Val(Sgnl)"=TRUE ("Value (Signaling)")) -> ()  [unwired: 2 in, 2 out]
          }
        }
      }
      event "Round T1 X": Value Change {
        n1194 = event-data() -> ()  [unwired: 7 out]
        n1195 = local read "BD 1 Frequency 1 (MHz)"() -> (w1864:dbl)
        n1196 = Round To Nearest(number=w1864) -> (nearest integer value=w1863:dbl)
        n1197 = property on="BD 1 Frequency 1 (MHz)" class="DigNum (strict)"("Val(Sgnl)"=w1863) -> ()  [unwired: 2 in, 2 out]
      }
      event "Round T2 X": Value Change {
        n1198 = event-data() -> ()  [unwired: 7 out]
        n1199 = local read "BD 1 Frequency 2 (MHz)"() -> (w1866:dbl)
        n1200 = Round To Nearest(number=w1866) -> (nearest integer value=w1865:dbl)
        n1201 = property on="BD 1 Frequency 2 (MHz)" class="DigNum (strict)"("Val(Sgnl)"=w1865) -> ()  [unwired: 2 in, 2 out]
      }
      event "Stop All": Value Change {
        n1202 = event-data() -> ()  [unwired: 7 out]
        n1203 = flat-sequence {
          tunnel: [w1871] -> w1870
          tunnel: [w1875] -> w1868
          tunnel: w1870 -> [w1875]
          tunnel: [TRUE] -> _
          tunnel: [w1873] -> w1869
          frame #0 {
            n1204 = call "hamilton_controller.vi"("action"=T42."DISCONNECT") -> ("error out"=w1871:errorcluster)  [unwired: 9 in, 1 out]
          }
          frame #1 {
            n1205 = local read "Stop All"() -> (w1873:bool)
          }
        }
      }
      event "Delayed Interlace Start": Value Change {
        n1206 = event-data() -> ()  [unwired: 7 out]
        n1207 = flat-sequence {
          frame #0 {
            n1208 = Multiply(x="Delay to Interlace (s)", y=1000.0) -> (x*y=w1877:dbl)
            n1209 = Wait (ms)(milliseconds to wait=w1877) -> ()  [unwired: 1 out]
          }
          frame #1 {
            n1210 = property on="Laser interlacing mode" class="RadioBtnsControl (strict)"("Val(Sgnl)"=enum32{"Laser ON", "Laser OFF", "Interlace"}."Interlace" ("Value (Signaling)")) -> ()  [unwired: 2 in, 2 out]
          }
        }
      }
      event "BD 1 Amplitude 1 (%)", "BD 1 Amplitude 2 (%)", "BD 1 Amplitude 3 (%)", "BD 2 Amplitude 1 (%)", "BD 2 Amplitude 2 (%)", "BD 2 Amplitude 3 (%)", "Trap 1 ON", "Trap 2 ON", "Trap 3 ON", "Feedback On/Off", "All FB On/Off": Value Change {
        w1902 = i16 1 ("f")
        n1211 = event-data() -> ()  [unwired: 7 out]
        n1212 = local write "Trap 1 (ON/OFF)"("Trap 1 ON") -> ()
        n1213 = local write "Trap 2 (ON/OFF)"("Trap 2 ON") -> ()
        n1214 = Boolean To (0,1)(Boolean="Trap 3 ON") -> (0, 1=w1903:i16)
        n1215 = Boolean To (0,1)(Boolean="Trap 1 ON") -> (0, 1=w1904:i16)
        n1216 = Boolean To (0,1)(Boolean="Trap 2 ON") -> (0, 1=w1905:i16)
        n1217 = Select(t=w1905, s="Trap ON/OFF X or Y Amp?", f=w1902) -> (s? t:f=w1900:i16)
        n1218 = Select(t=w1904, s="Trap ON/OFF X or Y Amp?", f=w1902) -> (s? t:f=w1901:i16)
        n1219 = Select(t=w1903, s="Trap ON/OFF X or Y Amp?", f=w1902) -> (s? t:f=w1899:i16)
        n1220 = Select(t=w1902, s="Trap ON/OFF X or Y Amp?", f=w1905) -> (s? t:f=w1897:i16)
        n1221 = Select(t=w1902, s="Trap ON/OFF X or Y Amp?", f=w1904) -> (s? t:f=w1898:i16)
        n1222 = Select(t=w1902, s="Trap ON/OFF X or Y Amp?", f=w1903) -> (s? t:f=w1896:i16)
        n1223 = And(x="All FB On/Off", y="Feedback On/Off") -> (x .and. y?=w1894:cluster{"Set 1":bool, "Set 2":bool})
        n1224 = local read "BD 1 Amplitude 1 (%)"() -> (w1912:dbl)
        n1225 = local read "BD 1 Amplitude 2 (%)"() -> (w1911:dbl)
        n1226 = local read "BD 1 Amplitude 3 (%)"() -> (w1910:dbl)
        n1227 = Unbundle By Name(w1894) -> ("Set 1"=w1889:bool, "Set 2"=w1886:bool)
        n1228 = local read "Y RF Amplitude Limits (%)"() -> (w1882:T24)
        n1229 = local read "X RF Amplitude Limits (%)"() -> (w1883:T24)
        n1230 = local read "BD 2 Amplitude 1 (%)"() -> (w1913:dbl)
        n1231 = local read "BD 2 Amplitude 2 (%)"() -> (w1914:dbl)
        n1232 = local read "BD 2 Amplitude 3 (%)"() -> (w1915:dbl)
        n1233 = And(x="Trap 2 ON", y=w1886) -> (x .and. y?=w1884:bool)
        n1234 = And(x="Trap 1 ON", y=w1889) -> (x .and. y?=w1887:bool)
        n1235 = Multiply(x=w1901, y=w1912) -> (x*y=w1909:dbl)
        n1236 = Multiply(x=w1911, y=w1900) -> (x*y=w1907:dbl)
        n1237 = Multiply(x=w1910, y=w1899) -> (x*y=w1908:dbl)
        n1238 = Multiply(x=w1913, y=w1898) -> (x*y=w1916:dbl)
        n1239 = Multiply(x=w1914, y=w1897) -> (x*y=w1917:dbl)
        n1240 = Multiply(x=w1915, y=w1896) -> (x*y=w1918:dbl)
        n1241 = call "set RF board amplitude - interlace.vi"("Board 2 Amplitude Limits"=w1882, "Board 1 Amplitude Limits"=w1883, "FPGA VI Reference In"=w1881, "Board 2 Amplitude 3 (%)"=w1918, "Board 1 Amplitude 3 (%)"=w1908, "Board 2 Amplitude 2 (%)"=w1917, "Board 2 Amplitude 1 (%)"=w1916, "Board 1 Amplitude 2 (%)"=w1907, "Board 1 Amplitude 1 (%)"=w1909) -> ("error out"=w1891:errorcluster, "FPGA VI Reference Out"=w1892:T36)  [unwired: 1 in]
        n1242 = xnode "Read/Write Control"("FPGA VI Reference In"=w1892, "error in"=w1891, "FB On/Off Set 1"=w1887, "FB On/Off Set 2"=w1884) -> ("error out"=w1890:errorcluster)  [unwired: 1 out]
      }
      event "Load parameters": Value Change {
        n1243 = event-data() -> ()  [unwired: 7 out]
        n1244 = property on="Saved AOD Raster Scan Parameter Sets" class="Arr (strict)"() -> ("Index Values"=w1929:u32[])  [unwired: 2 in, 2 out]
        n1245 = Index Array(array=w1929, index=0) -> (element=w1926:u32)
        n1246 = local write "Load parameters"(FALSE ("Load parameters")) -> ()
        n1247 = Index Array(array="Saved AOD Raster Scan Parameter Sets", index=w1926) -> (element=w1925:T46)
        n1248 = Unbundle By Name(w1925) -> ("Scan Range AOD (nm) 2"=w1924:dbl, "Step Size AOD (nm) 2"=w1923:dbl, "Scan Speed AOD (nm/s) 2"=w1922:dbl, "Number of scans (AOD) 2"=w1921:u16)
        n1249 = flat-sequence {
          tunnel: w1924 -> [w1932]
          tunnel: w1923 -> [w1931]
          tunnel: w1922 -> [w1930]
          tunnel: w1921 -> [w1933]
          frame #0 {
            n1250 = local write "Scan Speed (nm/s)"(w1930) -> ()
            n1251 = local write "Scan Range (nm)"(w1932) -> ()
            n1252 = local write "Step Size (nm)"(w1931) -> ()
          }
          frame #1 {
            n1253 = property on="Number of F/B Scans (AOD)" class="DigNum (strict)"("Val(Sgnl)"=w1933) -> ()  [unwired: 2 in, 2 out]
          }
        }
      }
      event "Trap 1 (ON/OFF)", "Trap 2 (ON/OFF)": Value Change {
        n1254 = event-data() -> ()  [unwired: 7 out]
        n1255 = flat-sequence {
          tunnel: [w1943] -> w1938
          tunnel: w1938 -> [w1958]
          tunnel: [w1944] -> w1934
          frame #0 {
            n1256 = local read "Trap 1 ON"() -> (w1943:bool)
          }
          frame #1 {
            n1257 = Exclusive Or(1:w1958, 2:"Trap 1 (ON/OFF)") -> (0:w1951:bool)
            n1258 = Select(t="on", s="Trap 2 (ON/OFF)", f="off") -> (s? t:f=w1950:string)
            n1259 = Select(t="on", s="Trap 1 (ON/OFF)", f="off") -> (s? t:f=w1946:string)
            n1260 = Build Array("trap 1 ", w1946) -> (w1945:string[])
            n1261 = Build Array("trap 2 " ("f"), w1950) -> (w1948:string[])
            n1262 = Select(t=w1945, s=w1951, f=w1948) -> (s? t:f=w1944:string[])
            n1263 = property on="Trap 1 ON" class="Bool (strict)"("Val(Sgnl)"="Trap 1 (ON/OFF)") -> ()  [unwired: 2 in, 2 out]
            n1264 = property on="Trap 2 ON" class="Bool (strict)"("Val(Sgnl)"="Trap 2 (ON/OFF)") -> ()  [unwired: 2 in, 2 out]
          }
        }
        n1265 = local read "Saving..."() -> (w1937:bool)
        n1266 = local read "Save Event Log?"() -> (w1936:bool)
        n1267 = And(x=w1937, y=w1936) -> (x .and. y?=w1935:bool)
        n1268 = case shown="True" w1935 {
          tunnel: w1934 -> [_ w1942]
          frame False {
          }
          frame True {
            n1269 = local read "Time (s)"() -> (w1939:dbl)
            n1270 = local read "log file ref"() -> (w1941:refnum<file>)
            n1271 = Concatenate Strings(w1942) -> (w1940:string)
            n1272 = call "write to event log.vi"("log file ref"=w1941, "time"=w1939, "input string"=w1940) -> ()  [unwired: 8 in]
          }
        }
      }
      event "DIO count 1 (ticks)", "DIO count 2 (ticks)", "DIO count 3 (ticks)", "Interlace", "Number Interlace Sets", "Not-Interlacing Set", "BD 1 Delay (ticks)", "BD 2 Delay (Ticks)", "Next trap write delay (ticks)", "XY phase ext loop method", "Amp switch delay 2", "BD 2 Delay (Ticks) 2", "BD 1 Delay (ticks) 2": Value Change {
        n1273 = event-data() -> ()  [unwired: 7 out]
        n1274 = To Unsigned Byte Integer(number="Not-Interlacing Set") -> (unsigned 8bit integer=w1959:u8)
        n1275 = Add(x=u8 1 ("y"), y=w1959) -> (x+y=w1968:u8)
        n1276 = local read "DIO count 1 (ticks)"() -> (w1975:u16)
        n1277 = local read "DIO count 2 (ticks)"() -> (w1974:u16)
        n1278 = local read "DIO count 3 (ticks)"() -> (w1973:u16)
        n1279 = xnode "Read/Write Control"("FPGA VI Reference In"=w1961, "DIO count 1 (ticks)"=w1975, "DIO count 2 (ticks)"=w1974, "DIO count 3 (ticks)"=w1973, "Interlace ON/OFF"="Interlace", "Number Interlace Cycles"="Number Interlace Sets", "Interlace Off Parameters"=w1968, "BD 1 Delay (ticks)"="BD 1 Delay (ticks)", "BD 2 Delay (Ticks)"="BD 2 Delay (Ticks)", "Next trap write delay (ticks)"="Next trap write delay (ticks)") -> ("error out"=w1977:errorcluster)  [unwired: 1 in, 1 out]
        n1280 = Build Array(w1975, w1974, w1973) -> (w1967:u16[])
        n1281 = Split 1D Array(array=w1967, index="Number Interlace Sets") -> (first subarray=w1976:u16[])  [unwired: 1 out]
        n1282 = Index Array(array=w1967, index=w1959) -> (element=w1966:u16)
        n1283 = Add Array Elements(numeric array=w1976) -> (sum=w1970:u16)
        n1284 = Select(t=w1970, s="Interlace", f=w1966) -> (s? t:f=→"Total Counts (ticks)":u16)
      }
      event "Reset Feedback": Value Change {
        n1285 = event-data() -> ()  [unwired: 7 out]
        n1286 = Unbundle By Name("Reset Feedback") -> ("Set 1"=w1981:bool, "Set 2"=w1980:bool)
        n1287 = xnode "Read/Write Control"("FPGA VI Reference In"=w1978, "FB Reset Set 1"=w1981, "FB Reset Set 2"=w1980) -> ("error out"=w1979:errorcluster)  [unwired: 1 in, 1 out]
      }
      event "Trap intensity output range", "Trap Intensity PID Gains": Value Change {
        n1288 = event-data() -> ()  [unwired: 7 out]
        n1289 = xnode "Read/Write Control"("FPGA VI Reference In"=w1985, "FB Gains"="Trap Intensity PID Gains", "FB output range"="Trap intensity output range") -> ("error out"=w1986:errorcluster)  [unwired: 1 in, 1 out]
      }
      event "AI2 to Setpoint", "Setpoints (V)": Value Change {
        n1290 = event-data() -> ()  [unwired: 7 out]
        n1291 = xnode "Read/Write Control"("FPGA VI Reference In"=w1987) -> ("FPGA VI Reference Out"=w1990:T36, "error out"=w1989:errorcluster, "AI2 Y Sum Set 1"=w1997:i16, "AI2 Y Sum Set 2"=w1996:i16)  [unwired: 1 in]
        n1292 = Cluster To Array(cluster="AI2 to Setpoint") -> (array=w2000:bool[])
        n1293 = local read "AI2 (V)"() -> (w1998:cluster{"Set 1":dbl, "Set 2":dbl})
        n1294 = Or Array Elements(Boolean array=w2000) -> (logical OR=w2001:bool)
        n1295 = Bundle By Name(cluster=w1998, "Set 1"=w1997, "Set 2"=w1996) -> (w1995:cluster{"Set 1":dbl, "Set 2":dbl})
        n1296 = Divide(x=w1995, y=3276.7) -> (x/y=w1994:cluster{"Set 1":dbl, "Set 2":dbl})
        "AI2 (V)" <- w1994
        n1297 = case shown="True" w2001 {
          tunnel: [w2004 w2021] -> w1993
          tunnel: "AI2 to Setpoint" -> [_ w2017]
          tunnel: "Setpoints (V)" -> [w2005 w2020]
          tunnel: w1994 -> [_ w2014]
          frame False {
            n1298 = Multiply(x=3276.7, y=w2005) -> (x*y=w2006:cluster{"Set 1":dbl, "Set 2":dbl})
            n1299 = To Word Integer(number=w2006) -> (16bit integer=w2004:cluster{"Set 1":i16, "Set 2":i16})
          }
          frame True {
            n1300 = Unbundle By Name(w2014) -> ("Set 1"=w2013:dbl, "Set 2"=w2012:dbl)
